vi "alignTo.vi"(6 "alignment":T1, 8 "error in (no error)":errorcluster, 10 "targetObj":refnum<class "GObject.lvclass">, 11 "GObject in":refnum<class "GObject.lvclass">) -> (0 "error out":errorcluster, 3 "GObject out":refnum<class "GObject.lvclass">)   [LabVIEW 2023, in "TLC_Scripto.lvlib" / "GObject.lvclass"]
uses:
  GObject.lvclass
  GObject.lvclass/GObject.ctl
  Ctrls/alignment.ctl
  TLC_Scripto.lvlib
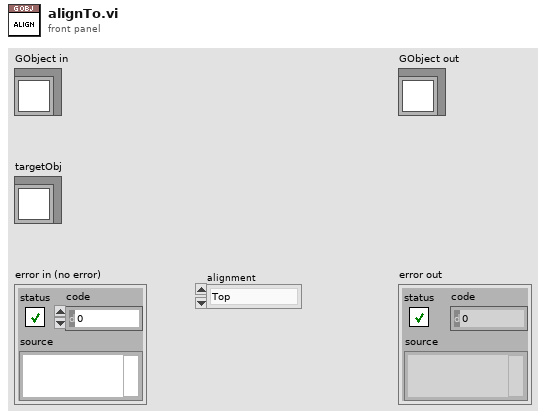
[diagram p1: front panel]
types:
  T1 = typedef "TLC_Scripto.lvlib/alignment.ctl" = enum16{"Top", "Bottom", "Left", "Right", "Center"}
  T2 = typedef "TLC_Scripto.lvlib/rectangle.ctl" = cluster{"left":i32, "top":i32, "right":i32, "bottom":i32}
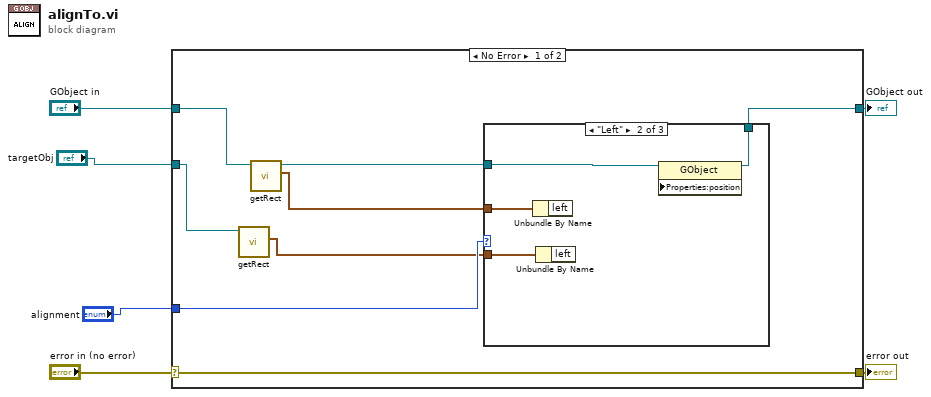
[diagram p0: block diagram]
diagram:
  n1 = case shown="No Error" "error in (no error)" {
    selector: "error in (no error)" -> [w14 w20]
    tunnel: [w14 w20] -> w5
    tunnel: [w7 w19] -> w3
    tunnel: "GObject in" -> [w9 w19]
    tunnel: "targetObj" -> [w13 _]
    tunnel: "alignment" -> [w12 _]
    frame No Error {
      n2 = call-dynamic "getRect.vi"("GObject in"=w13) -> ("rectangle"=w10:T2)  [unwired: 8 in, 2 out]
      n3 = call-dynamic "getRect.vi"("GObject in"=w9) -> ("rectangle"=w11:T2, "GObject out"=w8:refnum<class "GObject.lvclass">)  [unwired: 8 in, 1 out]
      n4 = case shown="\"Left\"" w12 {
        tunnel: w11 -> [_ w18 _]
        tunnel: w10 -> [_ w17 _]
        tunnel: w8 -> [_ w16 _]
        tunnel: [_ w15 _] -> w7
        frame "Top", Default {
        }
        frame "Left" {
          n5 = Unbundle By Name(w18) -> ()  [unwired: 1 out]
          n6 = Unbundle By Name(w17) -> ()  [unwired: 1 out]
          n7 = property class="GObject" props=["Properties:position"](reference=w16) -> (reference out=w15:refnum<class "GObject.lvclass">)  [unwired: 2 in, 1 out]
        }
        frame "Bottom" {
        }
      }
    }
    frame Error {
    }
  }
  "error out" <- w5
  "GObject out" <- w3
